vi "performQuack.vi"(8 "error in (no error)":errorcluster, 11 "Duck in":refnum<class "Duck.lvclass">) -> (0 "error out":errorcluster, 2 "State":string, 3 "Duck out":refnum<class "Duck.lvclass">)   [LabVIEW 2013, in "Duck.lvclass"]
uses:
  Duck.lvclass
  Duck.lvclass/Duck.ctl
  QuackBehavior/QuackBehavior.lvclass
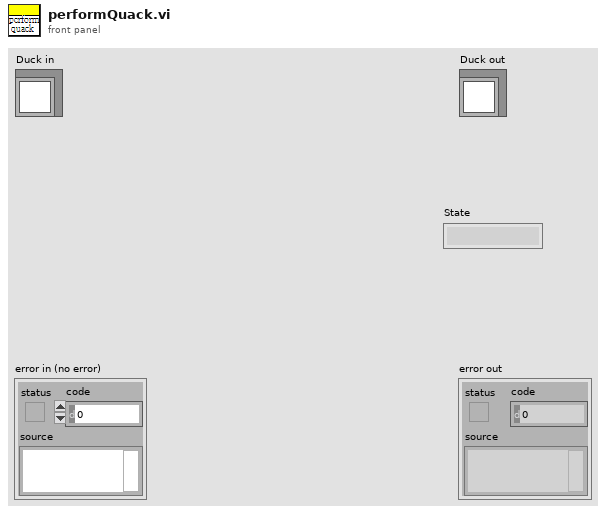
[diagram p1: front panel]
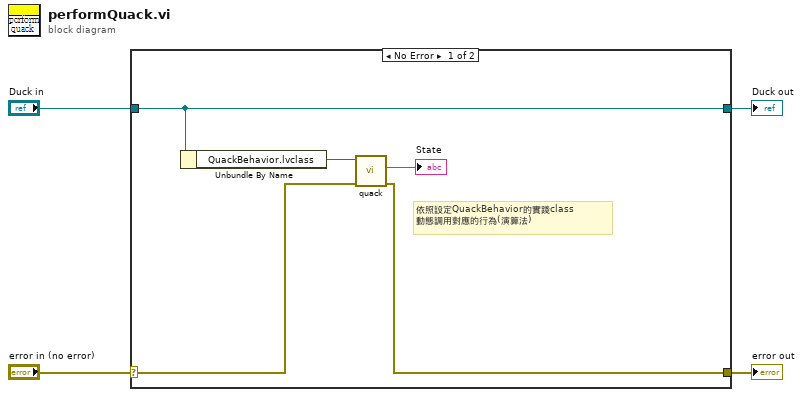
[diagram p0: block diagram]
diagram:
  n1 = case shown="No Error" "error in (no error)" {
    selector: "error in (no error)" -> [w7 w11]
    tunnel: [w5 w11] -> w3
    tunnel: [w9 w10] -> w1
    tunnel: "Duck in" -> [w9 w10]
    frame No Error {
      # "依照設定QuackBehavior的實踐class\n動態調用對應的行為(演算法)"
      n2 = Unbundle By Name(w9) -> ("QuackBehavior.lvclass"=w8:refnum<class "QuackBehavior.lvclass">)
      n3 = call-dynamic "quack.vi"("error in (no error)"=w7, "QuackBehavior in"=w8) -> ("error out"=w5:errorcluster, "String"=→"State":string)  [unwired: 7 in, 1 out]
    }
    frame Error {
    }
  }
  "error out" <- w3
  "Duck out" <- w1
